vi "CheckOneLvlibLinked.vi"(8 "error in (no error)":errorcluster, 10 "File Path to Append":path, 11 "Project Path":path=path "E:/sw-deps-monitor/Source/BuildSpecs/Modules/ModuleA.lvproj") -> (0 "error out":errorcluster)   [LabVIEW 2019, in "Hawkeye.lvlib"]
uses:
  Hawkeye.lvlib
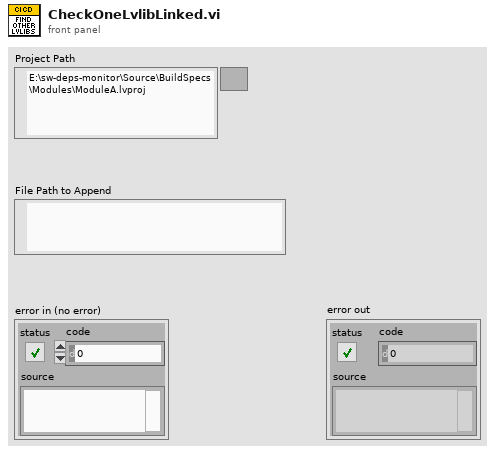
[diagram p1: front panel]
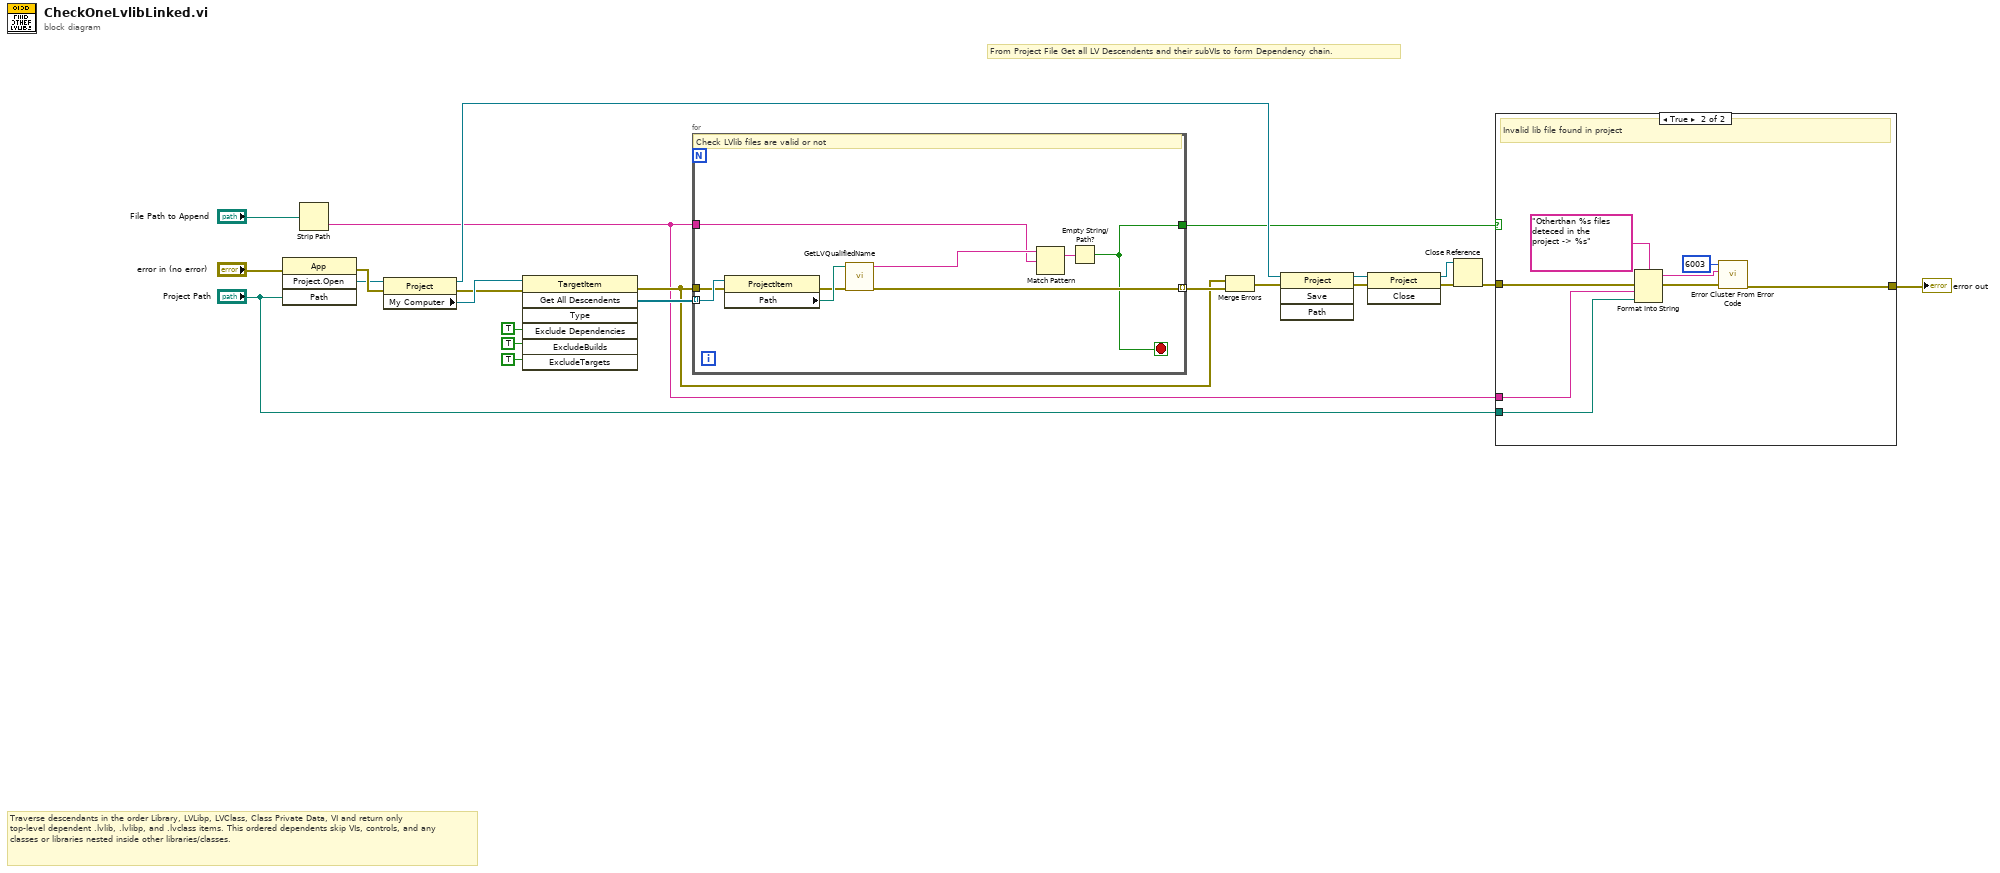
[diagram p0: block diagram]
diagram:
  # "From Project File Get all LV Descendents and their subVIs to form Dependency chain."
  # "Traverse descendants in the order Library, LVLibp, LVClass, Class Private Data, VI and return only top-level dependent .lvlib, .lvlibp, and .lvclass items. This ordered dependents skip VIs, controls, and any classes or libraries nested inside other libraries/classes."
  n1 = invoke class="App" method="Project.Open"(error in="error in (no error)", "Path"="Project Path") -> (error out=w23:errorcluster, "Project:Open"=w22:refnum<vi>)  [unwired: 2 in, 2 out]
  n2 = Strip Path(path="File Path to Append") -> (name=w5:string)  [unwired: 1 out]
  n3 = property class="Project"(reference=w22, error in=w23) -> (reference out=w15:refnum<vi>, error out=w17:errorcluster, "My Computer"=w18:refnum<vi>)
  n4 = invoke class="TargetItem" method="Get All Descendents"(reference=w18, error in=w17, "Exclude Dependencies"=TRUE ("ExcludeDependencies"), "ExcludeBuilds"=TRUE, "ExcludeTargets"=TRUE) -> (error out=w7:errorcluster, "All Descendents"=w9:refnum<vi>[])  [unwired: 2 in, 5 out]
  n5 = for {
    tunnel: w9 -> [w32] mode=indexing
    tunnel: w7 -> [w31]
    tunnel: [w28] -> w8 mode=indexing
    tunnel: w5 -> [w26]
    tunnel: [w24] -> w1
    stop <- w24 stop-if-true
    # "Check LVlib files are valid or not"
    n6 = property class="ProjectItem"(reference=w32, error in=w31) -> (error out=w29:errorcluster, "Path"=w30:path)  [unwired: 1 out]
    n7 = call "GetLVQualifiedName.vi"("error in (no error)"=w29, "LV File Path"=w30) -> ("error out"=w28:errorcluster, "VI Name / CTL Name / LVCLASS Name"=w27:string)  [unwired: 7 in, 1 out]
    n8 = Match Pattern(string=w27, regular expression=w26) -> (match substring=w25:string)  [unwired: 1 in, 3 out]
    n9 = Empty String/Path?(string/path=w25) -> (empty?=w24:bool)
  }
  n10 = Merge Errors(w7, w8) -> (w16:errorcluster)
  n11 = invoke class="Project" method="Save"(reference=w15, error in=w16) -> (reference out=w13:refnum<vi>, error out=w11:errorcluster)  [unwired: 2 in, 2 out]
  n12 = invoke class="Project" method="Close"(reference=w13, error in=w11) -> (reference out=w12:refnum<vi>, error out=w10:errorcluster)  [unwired: 1 in, 1 out]
  n13 = Close Reference(reference=w12, error in (no error)=w10) -> (error out=w3:errorcluster)
  n14 = case shown="True" w1 {
    tunnel: w5 -> [_ w37]
    tunnel: "Project Path" -> [_ w36]
    tunnel: w3 -> [w33 w35]
    tunnel: [w33 w34] -> w2
    frame False {
    }
    frame True {
      # "Invalid lib file found in project"
      n15 = Format Into String(format string="Otherthan %s files deteced in the project -> %s", error in=w35, w37, w36) -> (resulting string=w38:string, error out=w41:errorcluster)  [unwired: 1 in]
      n16 = call <vilib>:"Error Cluster From Error Code.vi"("error in (no error)"=w41, "error message (\"\")"=w38, "error code (0)"=6003) -> ("error out"=w34:errorcluster)  [unwired: 6 in]
    }
  }
  "error out" <- w2
